vi "zadSpr_001_PH.vi"() -> ()   [LabVIEW 2021]
panel:
  out "output cluster 1":T1
  out "cluster 2":T2
  in  "String":string="Drugi cluster"
  in  "Boolean":bool
  in  "Array":i16[](array[numeric])=[2020, 2021, 2020, 2020, 2020]
  in  "Cluster":T1={"Array"=[2020, 2020, 2020, 2020, 2020], "Boolean"=TRUE, "String"="pierwszy cluster"}
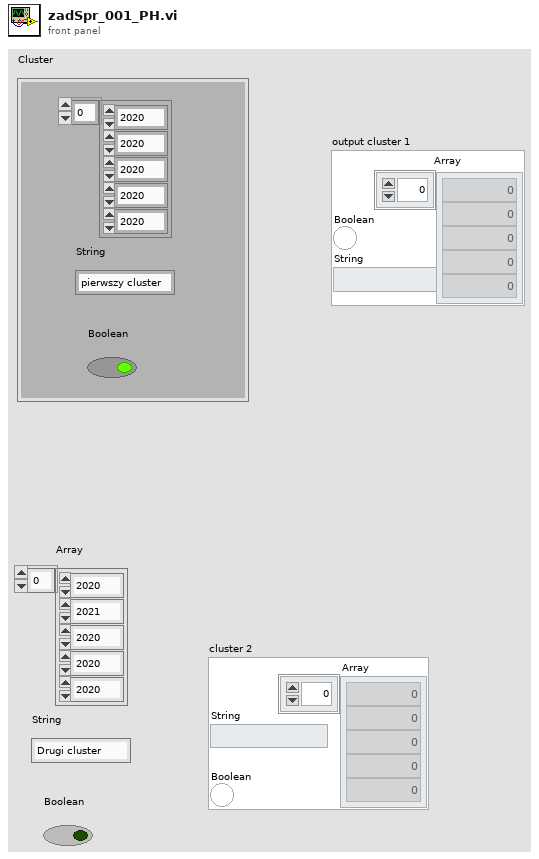
[diagram p1: front panel]
types:
  T1 = cluster{"Array":i16[], "Boolean":bool, "String":string}
  T2 = cluster{"Array":i16[], "String":string, "Boolean":bool}
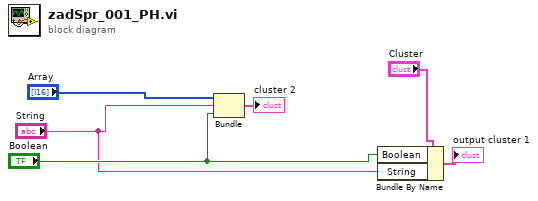
[diagram p0: block diagram]
diagram:
  n1 = Bundle("Array"="Array", "String"="String", "Boolean"="Boolean") -> (→"cluster 2":T2)  [unwired: 1 in]
  n2 = Bundle By Name(cluster="Cluster", "Boolean"="Boolean", "String"="String") -> (→"output cluster 1":T1)
